vi "set_autoscaling.vi"(8 "error in (no error)":errorcluster, 11 "DisplayDL090216 in":refnum<class "DisplayDL090216.lvclass">) -> (0 "error out":errorcluster, 3 "DisplayDL090216 out":refnum<class "DisplayDL090216.lvclass">)   [LabVIEW 2010, in "DisplayDL090216.lvclass"]
uses:
  DisplayDL090216.lvclass
  DisplayDL090216.lvclass/DisplayDL090216.ctl
  <vilib>/Utility/miscctls.llb/LVCursorListTypeDef.ctl
  <vilib>/Utility/miscctls.llb/LVPointDoubleTypeDef.ctl
  common/classes/ErrorController/ErrorController/class_data.vi
  common/classes/ErrorController/ErrorController/ErrorController.lvclass
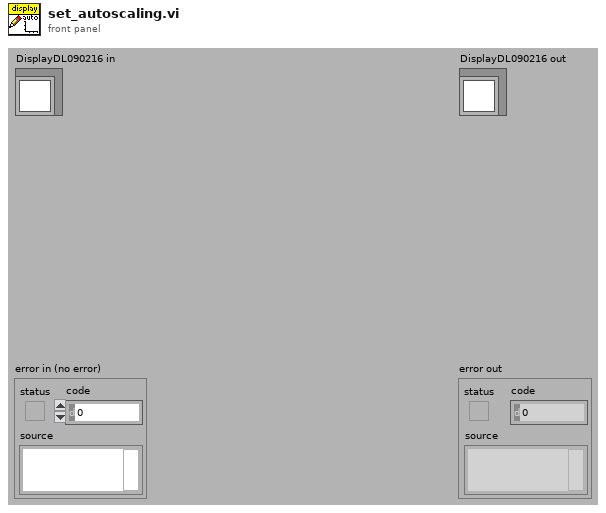
[diagram p1: front panel]
types:
  T1 = typedef "LVCursorListTypeDef.ctl" = cluster{"Name":string, "Color":u32, "Style":u8, "Point Style":u8, "Name Visible":bool, "Allow Drag":bool, "Cursor Mode":u32, "Plot":i32, "Index":i32, "Position":cluster{"X":dbl, "Y":dbl}, "X Scale":u32, "Y Scale":u32, "Watch Plots":i32[], "Watch All Plots":bool, "Plot Area":i32, "Label Offset":cluster{"X":dbl, "Y":dbl}}[]
  T2 = typedef "LVPointDoubleTypeDef.ctl" = cluster{"X":dbl, "Y":dbl}
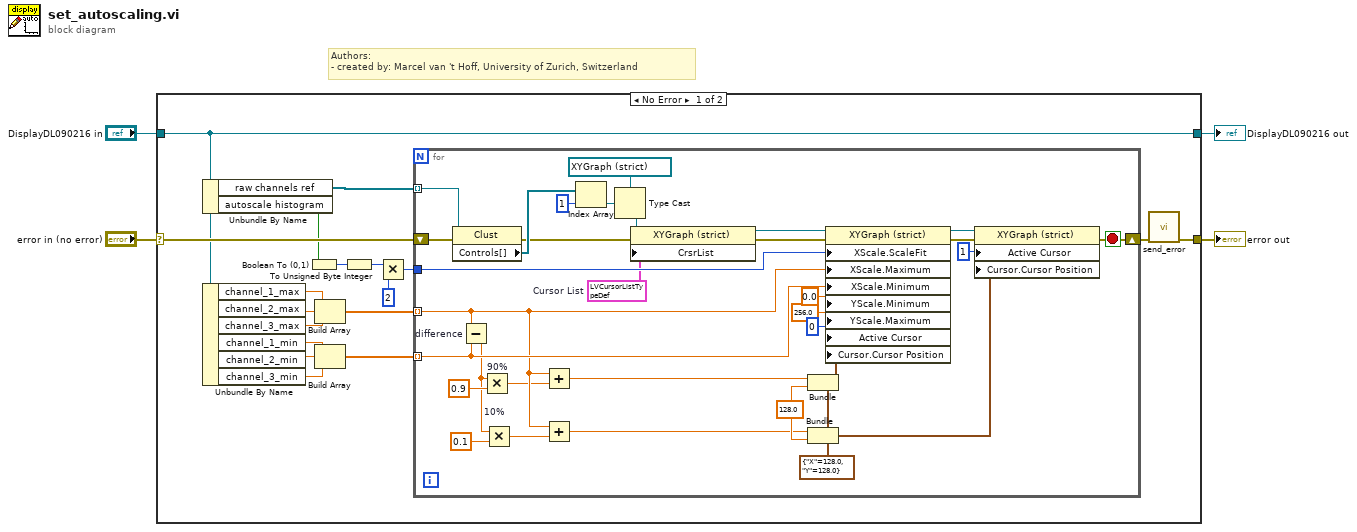
[diagram p0: block diagram]
diagram:
  # "Authors: \n- created by: Marcel van 't Hoff, University of Zurich, Switzerland"
  n1 = case shown="No Error" "error in (no error)" {
    selector: "error in (no error)" -> [w22 w56]
    tunnel: [w5 w56] -> w3
    tunnel: [w21 w55] -> w1
    tunnel: "DisplayDL090216 in" -> [w21 w55]
    frame No Error {
      n2 = Unbundle By Name(w21) -> ("raw channels ref"=w8:refnum<vi>[], "autoscale histogram"=w7:bool)
      n3 = Unbundle By Name(w21) -> ("channel_1_max"=w16:dbl, "channel_2_max"=w15:dbl, "channel_3_max"=w14:dbl, "channel_1_min"=w13:dbl, "channel_2_min"=w12:dbl, "channel_3_min"=w11:dbl)
      n4 = Boolean To (0,1)(Boolean=w7) -> (0, 1=w20:i16)
      n5 = Build Array(w16, w15, w14) -> (w10:dbl[])
      n6 = Build Array(w13, w12, w11) -> (w9:dbl[])
      n7 = To Unsigned Byte Integer(number=w20) -> (unsigned 8bit integer=w17:u8)
      n8 = Multiply(x=w17, y=u8 2) -> (x*y=w18:u8)
      n9 = for {
        tunnel: w8 -> [w54] mode=indexing
        shift-right: [w45] -> w6
        shift-left: w22 -> [w49]
        tunnel: w18 -> [w48]
        tunnel: w10 -> [w32] mode=indexing
        tunnel: w9 -> [w40] mode=indexing
        stop <- w45 stop-if-true
        w23 = T1 [{"Name"="Top saturation", "Color"=16711680, "Style"=5, "Point Style"=5, "Name Visible"=FALSE, "Allow Drag"=TRUE, "Cursor Mode"=1, "Plot"=-1, "Index"=115, "Position"={"X"=106495.675, "Y"=338.0}, "X Scale"=0, "Y Scale"=0, "Watch Plots"=[], "Watch All Plots"=FALSE, "Plot Area"=0, "Label Offset"={"X"=0.0, "Y"=-6.0}}, {"Name"="Bottom saturation", "Color"=4863, "Style"=5, "Point Style"=5, "Name Visible"=FALSE, "Allow Drag"=TRUE, "Cursor Mode"=1, "Plot"=-1, "Index"=52, "Position"={"X"=185684.76666666666, "Y"=369.0}, "X Scale"=0, "Y Scale"=0, "Watch Plots"=[], "Watch All Plots"=FALSE, "Plot Area"=0, "Label Offset"={"X"=0.0, "Y"=4.5}}]  # Cursor List
        w36 = T2 {"X"=128.0, "Y"=128.0} ("Cursor.Cursor Position")
        w35 = 128.0 ("Y Scale.Range:Minimum")
        n10 = property class="Clust"(reference=w54, error in=w49) -> (error out=w27:errorcluster, "Controls[]"=w53:refnum<vi>[])  [unwired: 1 out]
        n11 = Subtract "difference"(x=w32, y=w40) -> (x-y=w37:dbl)
        n12 = Multiply "90%"(x=w37, y=0.9) -> (x*y=w31:dbl)
        n13 = Multiply "10%"(x=w37, y=0.1) -> (x*y=w29:dbl)
        n14 = Add(x=w32, y=w31) -> (x+y=w30:dbl)
        n15 = Add(x=w32, y=w29) -> (x+y=w28:dbl)
        n16 = Index Array(array=w53, index=1) -> (element=w50:refnum<vi>)
        n17 = Type Cast(type=refnum<vi> refnum ("histogram out"), x=w50) -> (*(type *) &x=w25:refnum<vi>)
        n18 = property class="XYGraph (strict)"(reference=w25, error in=w27, "CrsrList"=w23) -> (reference out=w24:refnum<vi>, error out=w26:errorcluster)
        n19 = Bundle(cluster=w36, "X"=w30, "Y"=w35) -> (w34:T2)
        n20 = Bundle(cluster=w36, "X"=w28, "Y"=w35) -> (w33:T2)
        n21 = property class="XYGraph (strict)"(reference=w24, error in=w26, "XScale.ScaleFit"=w48, "XScale.Maximum"=w32, "XScale.Minimum"=w40, "YScale.Minimum"=0.0 ("Y Scale.Range:Minimum"), "YScale.Maximum"=256.0 ("Y Scale.Range:Maximum"), "Active Cursor"=u32 0, "Cursor.Cursor Position"=w34) -> (reference out=w47:refnum<vi>, error out=w46:errorcluster)
        n22 = property class="XYGraph (strict)"(reference=w47, error in=w46, "Active Cursor"=u32 1, "Cursor.Cursor Position"=w33) -> (error out=w45:errorcluster)  [unwired: 1 out]
      }
      n23 = call "send_error.vi"("error in (no error)"=w6) -> ("error out"=w5:errorcluster)  [unwired: 10 in]
    }
    frame Error {
    }
  }
  "error out" <- w3
  "DisplayDL090216 out" <- w1
